vi "set gain attempt 1.vi"(8 "error in (no error)":errorcluster, 10 "Gain":dbl=50.0, 11 "VISA resource name":refnum<visa-resource-name>="GPIB0::12::INSTR") -> (0 "error out":errorcluster, 3 "VISA resource name out":refnum<visa-resource-name>)   [LabVIEW 2009]
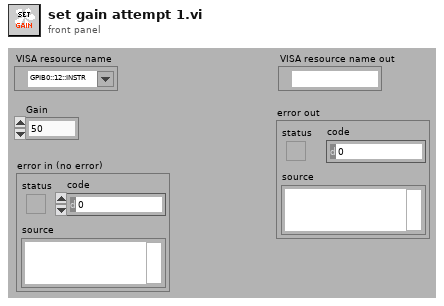
[diagram p1: front panel]
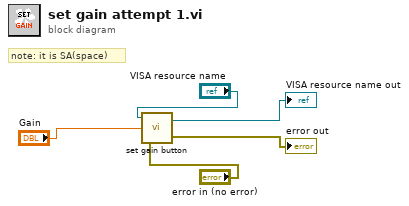
[diagram p0: block diagram]
diagram:
  # "note: it is SA(space)"
  n1 = call "set gain button.vi"("error in (no error)"="error in (no error)", "Gain"="Gain", "VISA resource name"="VISA resource name") -> ("error out"=→"error out":errorcluster, "VISA resource name out"=→"VISA resource name out":refnum<visa-resource-name>)
